vi "TestArmPathPlanner.vi"() -> ()   [LabVIEW 2018]
uses:
  TypeDefs/ArmAbsolutePosition.ctl
  General/MotionProfiling/TypeDefs/MotionProfileGeneratorParams.ctl
  <vilib>/Rock Robotics/WPI/ThirdParty/Phoenix-LabVIEW/Motor Controller/Controls/CTRE_Phoenix_MotorControl_TrajectoryPointTimeDur.ctl
  TypeDefs/ArmPassThroughParams.ctl
  TypeDefs/RobotID.ctl
  ArgosLib/Path Planning/TypeDefs/Point2D.ctl
  General/MotionProfiling/TypeDefs/TrajectoryPoint.ctl
  ArgosLib/ArgosLib.lvlib
panel:
  in  "PathPercent":dbl(slide) min=0.0 max=1.0 scale=0.0..1.0
  out "Arm Position":cluster{"X":dbl[], "Y":dbl[]}[](graph)=[{"X"=[-15.5, -15.5, -6.0, -6.0, 6.0, 6.0, 15.5, 15.5, 45.5, 45.5, 6.0, 6.0, -6.0, -6.0, -45.5, -45.5, -15.5], "Y"=[0.0, 7.0, 7.0, 12.0, 12.0, 7.0, 7.0, 0.0, 0.0, 90.0, 90.0, 24.0, 24.0, 90.0, 90.0, 0.0, 0.0]}, {"X"=array[361 elements], "Y"=array[361 elements]}, {"X"=array[361 elements], "Y"=array[361 elements]}, {"X"=[0.0, 21.000000000000004], "Y"=[44.25, 15.0]}, {"X"=[21.000000000000004, 26.99999809759101], "Y"=[15.0, 14.995222039735602]}, {"X"=[22.499999524397754, 22.499999524397758, 19.500000475602256, 19.500000475602253], "Y"=[14.9988055099339, 2.9988055099339004, 3.0011944900660996, 15.0011944900661]}]
  in  "Arm Pass Through Params":T1={"Pass Through Length (in)"=12.0, "Pass Through Min Height (in)"=12.0, "Pass Through Max Height (in)"=24.0, "Pass Through Wrist Angle (rad)"=0.0}
  out "Arm Wrist":T2(graph)={0.0, "Trajectory Point Interval (ms)"=40, [[4.055897027348257, 4.0550953656373006, 4.052237232134716, 4.04613843318791, 4.034997591857871, 4.015899135122442, 3.9848675439678005, 3.9367206365092895, 3.8639563502761987, 3.755694393958681, 3.5953226370164195, 3.360426119927916, 2.9841364514203983, 2.5860313232788723, 2.1668910532018417, 1.7245198623311084, 1.2463662836528413, 0.7434064615242622, 0.3302693816975075, 0.08764821007316621, -0.19010567504352455, -0.4928479002364374, -0.8053552192393434, -1.2552038154588934, -1.758124246438066, -2.287000533586975, -2.8485912983693416, -3.4544278992698296, -3.9992385919893625, -4.477495883282476, -4.902108995690553, -5.245537269018449, -5.245537269018449, -5.245537269018449, -5.245537269018449, -5.245537269018449, -5.245537269018449, -5.245537269018449, -5.245537269018449, -5.245537269018449, -5.245537269018449], [163.54485136741283, -0.020041542773907572, -0.0714533375646198, -0.15246997367013293, -0.2785210332509891, -0.4774614183857162, -0.7757897788660428, -1.2036726864627756, -1.819107155827271, -2.7065489079379446, -4.009293923556534, -5.872412927212589, -9.407241712687942, -9.952628203538149, -10.478506751925764, -11.059279771768331, -11.953839466956678, -12.573995553214479, -10.328426995668865, -6.065529290608533, -6.943847127917269, -7.5685556298228205, -7.81268297507265, -11.246214905488749, -12.573010774479314, -13.221907178722725, -14.039769119559164, -15.145915022512202, -13.620267317988322, -11.956432282327834, -10.615327810201935, -8.585706833197392, 0.0, 0.0, 0.0, 0.0, 0.0, 0.0, 0.0, 0.0, 0.0], [4088.6212841853207, -4089.122322754668, -1.2852948697678057, -2.0254159026378282, -3.151276489521404, -4.973509628368178, -7.458209012008165, -10.697072689918318, -15.385861734112382, -22.18604380276684, -32.56862539046473, -46.57797509140138, -88.3707196368838, -13.634662271255182, -13.146963709690374, -14.519325496064184, -22.363992379708673, -15.503902156445015, 56.13921393864034, 106.57244262650829, -21.95794593271838, -15.617712547638796, -6.103183631245734, -85.83829826040248, -33.169896724764136, -16.22241010608527, -20.446548520910966, -27.653647573825957, 38.141192613097004, 41.595875891512215, 33.52761180314747, 50.74052442511356, 214.6426708299348, 0.0, 0.0, 0.0, 0.0, 0.0, 0.0, 0.0, 0.0]]}
  out "Arm Shoulder":T2(graph)={0.0, "Trajectory Point Interval (ms)"=40, [[-2.485897027348257, -2.4851072958162197, -2.4823169806359386, -2.476610959105788, -2.466857228156793, -2.4515085113917974, -2.4287729667025824, -2.3963527600398518, -2.350431137808563, -2.284513709864505, -2.187157401405465, -2.040243693099315, -1.786824197239345, -1.5209887802060515, -1.2482788401614453, -0.9732781561615349, -0.6982771787555206, -0.4515858882028595, -0.3049850740385021, -0.10226983612994925, 0.11683754563303896, 0.3154399571329603, 0.4793394777948856, 0.7278750207432971, 1.0028758829523126, 1.2778768678302974, 1.5482951319817302, 1.8072546515485026, 1.9888767348636507, 2.1090685590963103, 2.1917192749834253, 2.2455372690184494, 2.2455372690184494, 2.2455372690184494, 2.2455372690184494, 2.2455372690184494, 2.2455372690184494, 2.2455372690184494, 2.2455372690184494, 2.2455372690184494, 2.2455372690184494], [0.0, 0.01974328830093297, 0.06975787950702639, 0.1426505382537635, 0.24384327372487524, 0.38371791912489295, 0.5683886172303754, 0.810505166568265, 1.1480405557822149, 1.6479356986014548, 2.433907711476002, 3.672842707653745, 6.335487396499251, 6.645885425832337, 6.817748501115156, 6.87501709999776, 6.875024435150356, 6.167282263816529, 3.6650203541089343, 5.067880947713822, 5.477684544074705, 4.965060287498034, 4.097488016548133, 6.213388573710287, 6.875021555225386, 6.875024621949621, 6.760456603785819, 6.473987989169311, 4.540552082878701, 3.0047956058164904, 2.066267897177876, 1.3454498508756019, 0.0, 0.0, 0.0, 0.0, 0.0, 0.0, 0.0, 0.0, 0.0], [0.0, 0.49358220752332427, 1.2503647801523354, 1.822316468668428, 2.5298183867777935, 3.4968661350004426, 4.616767452637061, 6.05291373344724, 8.438384730348746, 12.497378570480999, 19.649300321863684, 30.973374904443574, 66.56611722113765, 7.759950733327159, 4.29657688207048, 1.4317149720650901, 0.0001833788149108173, -17.69355428334569, -62.55654774268986, 35.071514840122184, 10.245089909022086, -12.815606414416791, -21.689306773747518, 52.897513929053865, 16.540824537877462, 7.666810588613515e-05, -2.864200454095056, -7.161715365412702, -48.33589765726525, -38.39391192655527, -23.463192715965363, -18.02045115755685, -33.636246271890045, 0.0, 0.0, 0.0, 0.0, 0.0, 0.0, 0.0, 0.0]]}
  out "Arm Extension":T2(graph)={0.0, "Trajectory Point Interval (ms)"=40, [[32.80243893371346, 32.73382329193226, 32.493830843461815, 32.014621982811256, 31.229704827724923, 30.07518621108094, 28.525539440458076, 26.595412909760075, 24.309668612420545, 21.71207960984723, 18.884301063490575, 16.058129522650766, 15.999999999999998, 15.999999999999998, 15.999999999999998, 15.999999999999998, 15.999999999999998, 17.018325645108163, 20.46619395704584, 20.10504894569543, 20.137290914005387, 20.263349380795905, 17.08862745921232, 15.999999999999998, 15.999999999999998, 15.999999999999998, 15.999999999999998, 15.999999999999998, 18.22509445834179, 20.899787030356347, 23.467846205438114, 25.612496949731394, 25.612496949731394, 25.612496949731394, 25.612496949731394, 25.612496949731394, 25.612496949731394, 25.612496949731394, 25.612496949731394, 25.612496949731394, 25.612496949731394], [0.0, -1.7153910445300014, -5.999811211761141, -11.980221516263967, -19.62292887715833, -28.862965416099584, -38.74116926557161, -48.25316326745001, -57.14360743348825, -64.93972506433288, -70.69446365891636, -70.65428852099522, -1.4532380662692024, 0.0, 0.0, 0.0, 0.0, 25.458141127704124, 86.19670779844188, -9.028625283760228, 0.8060492077489378, 3.151461669762945, -79.36804803958965, -27.21568648030801, 0.0, 0.0, 0.0, 0.0, 55.62736145854479, 66.86731430036392, 64.2014793770442, 53.616268607331996, 0.0, 0.0, 0.0, 0.0, 0.0, 0.0, 0.0, 0.0, 0.0], [0.0, -42.884776113250034, -107.11050418077849, -149.51025761257063, -191.06768402235906, -231.00091347353134, -246.95509623680056, -237.79985004696016, -222.2611041509559, -194.90294077111568, -143.86846486458714, 1.0043784480284756, 1730.0262613681502, 36.33095165673006, 0.0, 0.0, 0.0, 636.4535281926031, 1518.4641667684439, -2380.6333270550526, 245.86686228772913, 58.635311550350174, -2062.987742733815, 1303.809038982041, 680.3921620077002, 0.0, 0.0, 0.0, 1390.6840364636198, 280.9988210454781, -66.64587308299303, -264.63026924280496, -1340.4067151832999, 0.0, 0.0, 0.0, 0.0, 0.0, 0.0, 0.0, 0.0]]}
  out "Overall Motion":T2(graph)={0.0, "Trajectory Point Interval (ms)"=40, [[0.0, 0.07333333333333872, 0.32999999999999285, 0.8433333333333345, 1.6866666666666708, 2.933333333333337, 4.6200000000000045, 6.7466666666666715, 9.313333333333336, 12.320000000000004, 15.766666666666662, 19.577263128138455, 23.628890034857097, 27.882256707389793, 32.24561574810349, 36.645626692102056, 41.045642330598284, 45.23180493891788, 49.631804938917895, 53.752665022664445, 58.15266502266445, 62.15987106543, 66.55987106542999, 70.80102207008076, 75.20103586542501, 79.60105162347277, 83.92774384989569, 88.07109616296405, 91.88469944610591, 95.44136611277257, 98.59469944610589, 101.11264147745605, 101.11264147745605, 101.11264147745605, 101.11264147745605, 101.11264147745605, 101.11264147745605, 101.11264147745605, 101.11264147745605, 101.11264147745605, 101.11264147745605], [0.0, 1.8333333333334678, 6.416666666666354, 12.83333333333354, 21.083333333333407, 31.166666666666657, 42.166666666666686, 53.16666666666667, 64.16666666666661, 75.16666666666669, 86.16666666666646, 95.26491153679481, 101.29067266796605, 106.3341668133174, 109.0839760178424, 110.00027359996416, 110.0003909624057, 104.65406520798996, 110.00000000000031, 103.02150209366374, 110.00000000000014, 100.18015106913882, 109.9999999999996, 106.02877511626936, 110.00034488360626, 110.00039395119394, 108.16730566057302, 103.58380782670906, 95.34008207854647, 88.91666666666644, 78.83333333333304, 62.94855078375399, 0.0, 0.0, 0.0, 0.0, 0.0, 0.0, 0.0, 0.0, 0.0], [0.0, 45.8333333333367, 114.58333333332216, 160.41666666667965, 206.24999999999667, 252.08333333333127, 275.0000000000007, 274.99999999999966, 274.9999999999986, 275.00000000000176, 274.9999999999943, 227.45612175320886, 150.64402827928092, 126.08735363378365, 68.74523011312519, 22.90743955304393, 0.002934061038573077, -133.6581438603936, 133.64836980025885, -174.46244765841428, 174.46244765841, -245.49622327153315, 245.49622327151965, -99.2806220932561, 99.28924418342255, 0.0012266896920465342, -45.82720726552303, -114.58744584659897, -206.09314370406472, -160.58538529700073, -252.083333333335, -397.1195637394764, -1573.7137695938497, 0.0, 0.0, 0.0, 0.0, 0.0, 0.0, 0.0, 0.0]]}
  out "TravelTime (s)":dbl
  in  "MotionProfileGeneratorParameters":T3={"Trajectory Point Interval (ms)"=40, "Maximum Travel Speed (units/s)"=110.0, "Velocity Ramp Time (ms)"=400.0, "Acceleration Ramp Time (ms)"=200.0} {"Acceleration Ramp Time (ms)" min=1.0; "Velocity Ramp Time (ms)" min=1.0; "Maximum Travel Speed (units/s)" min=0.0; "Trajectory Point Interval (ms)" items=["TrajectoryDuration_0ms"=0, "TrajectoryDuration_5ms"=5, "TrajectoryDuration_10ms"=10, "TrajectoryDuration_20ms"=20, "TrajectoryDuration_30ms"=30, "TrajectoryDuration_40ms"=40, "TrajectoryDuration_50ms"=50, "TrajectoryDuration_100ms"=100]}
  in  "EndPoint":T5={"X (in)"=21.0, "Y (in)"=15.0, "Wrist (rad)"=1.57}
  in  "StartPoint":T5={"X (in)"=-18.0, "Y (in)"=50.0, "Wrist (rad)"=-1.0}
  in  "PathPointSpacing (in)":dbl=0.25
  out "PathLength (in)":dbl
  out "NumPoints":i32
  out "Path":cluster{dbl[], dbl[]}[](graph)=[{array[361 elements], array[361 elements]}, {array[361 elements], array[361 elements]}, {[-15.5, -15.5, -6.0, -6.0, 6.0, 6.0, 15.5, 15.5, 45.5, 45.5, 6.0, 6.0, -6.0, -6.0, -45.5, -45.5, -15.5], [0.0, 7.0, 7.0, 12.0, 12.0, 7.0, 7.0, 0.0, 0.0, 90.0, 90.0, 24.0, 24.0, 90.0, 90.0, 0.0, 0.0]}, {[-17.999999999999996, -17.969269066986136, -17.861710801437624, -17.64659427034059, -17.293188540681186, -17.23694880570164, -17.447845453869164, -17.482830899137877, -17.18187066722039, -16.361013245924966, -14.82948179588336, -12.47007247741721, -9.304518318749695, -6.95514637829422, -3.8898652435061973, 0.5101347564938068, 4.836801423160476, 8.558633631835997, 11.891422803105423, 14.941239308889699, 17.645200334636595, 19.97186447306996, 21.000000000000004, 21.000000000000004, 21.000000000000004, 21.000000000000004, 21.000000000000004, 21.000000000000004, 21.000000000000004, 21.000000000000004, 21.000000000000004], [50.0, 49.9334163118033, 49.70037340311485, 49.23428758573795, 48.468575171475905, 47.27284565759164, 45.60007000481347, 43.47500080506513, 40.928355772375475, 38.03974673892701, 34.95825798541716, 31.972081104358047, 29.42853115052185, 26.06948381963748, 24.0, 23.999999999999993, 23.999999999999993, 22.464819820898406, 20.465146318136746, 18.635256414666177, 17.01287979921804, 15.616881316158025, 15.0, 15.0, 15.0, 15.0, 15.0, 15.0, 15.0, 15.0, 15.0]}]
  out "Update Rate (Hz)":dbl
  in  "stop":bool
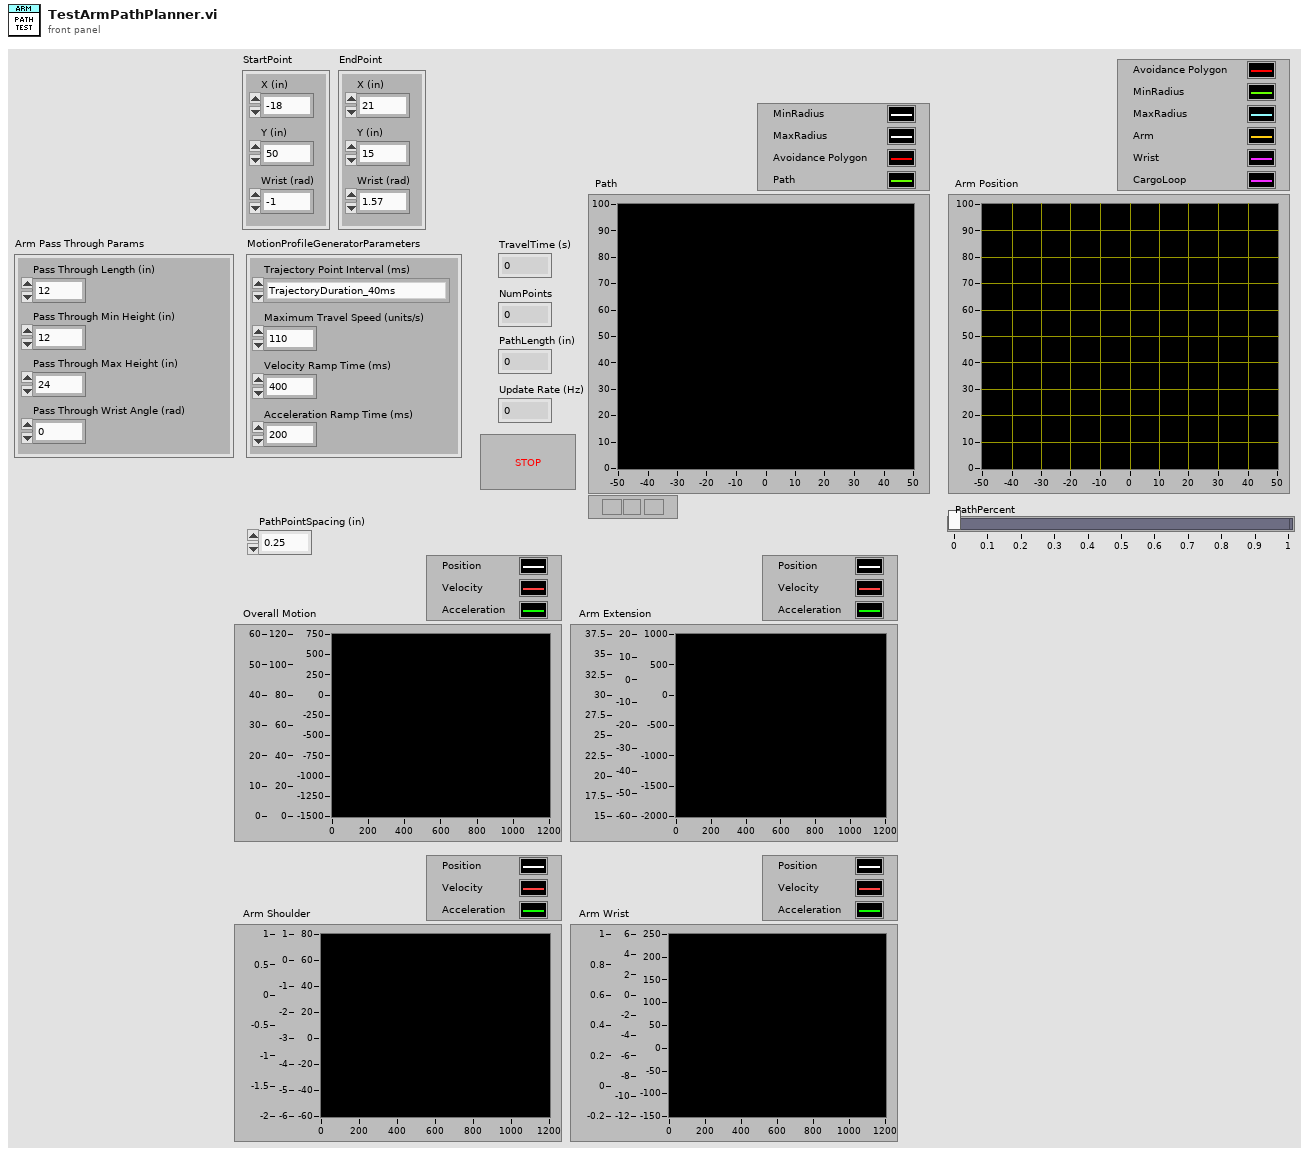
[diagram p1: front panel]
types:
  T1 = typedef "ArmPassThroughParams.ctl" = cluster{"Pass Through Length (in)":dbl, "Pass Through Min Height (in)":dbl, "Pass Through Max Height (in)":dbl, "Pass Through Wrist Angle (rad)":dbl}
  T2 = cluster{dbl, "Trajectory Point Interval (ms)":i32, dbl[][]}
  T3 = typedef "MotionProfileGeneratorParams.ctl" = cluster{"Trajectory Point Interval (ms)":T4, "Maximum Travel Speed (units/s)":dbl, "Velocity Ramp Time (ms)":dbl, "Acceleration Ramp Time (ms)":dbl}
  T4 = typedef "CTRE_Phoenix_MotorControl_TrajectoryPointTimeDur.ctl" = i32
  T5 = typedef "ArmAbsolutePosition.ctl" = cluster{"X (in)":dbl, "Y (in)":dbl, "Wrist (rad)":dbl}
  T6 = typedef "ArgosLib.lvlib/Point2D.ctl" = cluster{"X (in)":dbl, "Y (in)":dbl}
  T7 = typedef "RobotID.ctl" = enum16{"Competition", "Practice", "Programming"}
  T8 = typedef "TrajectoryPoint.ctl" = cluster{"Position ":dbl, "Velocity ":dbl, "Time (ms)":T4, "Last Point":bool}
  T9 = typedef "Config_Robot.ctl" = cluster{"Motors":cluster{"DriveRightPrimary":T10, "DriveRightSecondary":T10, "DriveLeftPrimary":T10, "DriveLeftSecondary":T10, "RearClimb":T10, "Front Climb":T10, "Climb Drive":T10, "Shoulder1":T10, "Shoulder2":T10, "Wrist":T10, "Extension":T10, "CargoIntake":T10, "Intake2":T10}, "Sensors":cluster{"IMU":T15, "HomingButton":T17, "HomingLED_Green":T17, "HomingLED_Yellow":T17, "HomingLED_Red":T17}, "PID":cluster{"FrontClimb":T19, "RearClimb":T19, "ArmShoulder":T19, "ArmExtend":T19, "ArmWrist":T19}, "Solenoids":cluster{" Shifter":T20, "Hatch Grip":T20, "Hatch Extend":T20, "Manipulator Slide":T20, "Hatch Floor Intake":T20}, "Enable Compressor":bool, "MotionMagic":cluster{"FrontClimbExtend":T22, "RearClimbExtend":T22, "FrontClimbRetract":T22, "RearClimbRetract":T22}, "RobotDimensions":T23, "Arm Home Position":T24, "Climb Home Position":cluster{"Back Climb":dbl, "Front Climb":dbl}, "Climb Positions":T25}
  T10 = typedef "ArgosLib.lvlib/Config_Motor.ctl" = cluster{"CAN Address":u8, "Invert":bool, "InvertSensor":bool, "Unit Conversion Factor":dbl, "Brake Mode":T11, "Reverse Limt Switch Mode":T12, "Forward Limt Swith Mode":T12, "PWM Channel":T13, "Motor Controller Type":T14, "Peak Current (A)":i32, "Continuos Current (A)":i32, "Peak Duration (ms)":i32, "Current Limit Enable":bool}
  T11 = typedef "CTRE_Phoenix_MotorControl_NeutralMode.ctl" = enum8{"EEPROMSetting", "Override to Coast", "Override to Brake"}
  T12 = typedef "CTRE_Phoenix_MotorControl_LimitSwitchNormal.ctl" = enum16{"Normally Open", "Normally Closed", "Disabled"}
  T13 = typedef "FPGA_DIOPWMChannel.ctl" = enum8{"PWM 0", "PWM 1", "PWM 2", "PWM 3", "PWM 4", "PWM 5", "PWM 6", "PWM 7", "PWM 8", "PWM 9", "PWM MXP 0", "PWM MXP 1", "PWM MXP 2", "PWM MXP 3", "PWM MXP 4", "PWM MXP 5", "PWM MXP 6", "PWM MXP 7", "PWM MXP 8", "PWM MXP 9", "Invalid"}
  T14 = typedef "ArgosLib.lvlib/Config_MotorCtrlType.ctl" = enum16{"Disabled", "Talon SRX", "Talon SR"}
  T15 = typedef "ArgosLib.lvlib/Config_IMU.ctl" = cluster{"Yaw Axis":enum16{"X", "Y", "Z"}, "SPI Bus":T16, "AHRS Algorithm":enum16{"Complementary", "Madgwick"}, "Calibration Time (s)":dbl, "Calibrate On Open":bool}
  T16 = typedef "spi_bus.ctl" = enum16{"SPI On-Board, CS0", "SPI On-Board, CS1", "SPI On-Board, CS2", "SPI On-Board, CS3", "SPI MXP", "Invalid"}
  T17 = typedef "ArgosLib.lvlib/Config_DigitalIO.ctl" = cluster{"DIOChannel":T18, "Active Low":bool}
  T18 = typedef "FPGA_DIOChannel.ctl" = enum8{"DIO 0", "DIO 1", "DIO 2", "DIO 3", "DIO 4", "DIO 5", "DIO 6", "DIO 7", "DIO 8", "DIO 9", "DIO MXP 0", "DIO MXP 1", "DIO MXP 2", "DIO MXP 3", "DIO MXP 4", "DIO MXP 5", "DIO MXP 6", "DIO MXP 7", "DIO MXP 8", "DIO MXP 9", "DIO MXP 10", "DIO MXP 11", "DIO MXP 12", "DIO MXP 13", "DIO MXP 14", "DIO MXP 15", "SPI Port CS1", "SPI Port CS2", "SPI Port CS3", "SPI Port MISO", "SPI Port MOSI", "Invalid"}
  T19 = typedef "ArgosLib.lvlib/Config_PIDParams.ctl" = cluster{"P":dbl, "I":dbl, "D":dbl, "F":dbl, "IZone":dbl}
  T20 = typedef "ArgosLib.lvlib/Config_SingleSolenoid.ctl" = cluster{"SolenoidChannel":T21, "Invert":bool}
  T21 = typedef "WPI_SolenoidChannel.ctl" = enum8{"Solenoid 0", "Solenoid 1", "Solenoid 2", "Solenoid 3", "Solenoid 4", "Solenoid 5", "Solenoid 6", "Solenoid 7", "Invalid"}
  T22 = typedef "Config_MotionMagicParams.ctl" = cluster{"CruiseVelocity":i32, "Acceleration":i32}
  T23 = typedef "Config_Dimensions.ctl" = cluster{"Length (in)":dbl, "Shoulder Height (in)":dbl, "Frame Height (in)":dbl, "Arm Center to Front of Robot (in)":dbl, "Arm Min Extension (in)":dbl, "Arm Max Extension (in)":dbl, "Cargo Intake Loop Length (in)":dbl, "Cargo Intake Loop Width (in)":dbl, "Cargo Intake Loop Offset (in)":dbl, "Cargo Intake Loop Angle (rad)":dbl}
  T24 = typedef "ArmCoordinate.ctl" = cluster{"Radius (in)":dbl, "ShoulderAngle (rad)":dbl, "WristAngle (rad)":dbl}
  T25 = typedef "ClimberPositionHeights.ctl" = cluster{"Retract":dbl, "Level 2":dbl, "Level 3":dbl}
  T26 = typedef "ArgosLib.lvlib/Polygon2D.ctl" = T6[]
  T27 = cluster{dbl, "Trajectory Point Interval (ms)":T4, dbl[][]}
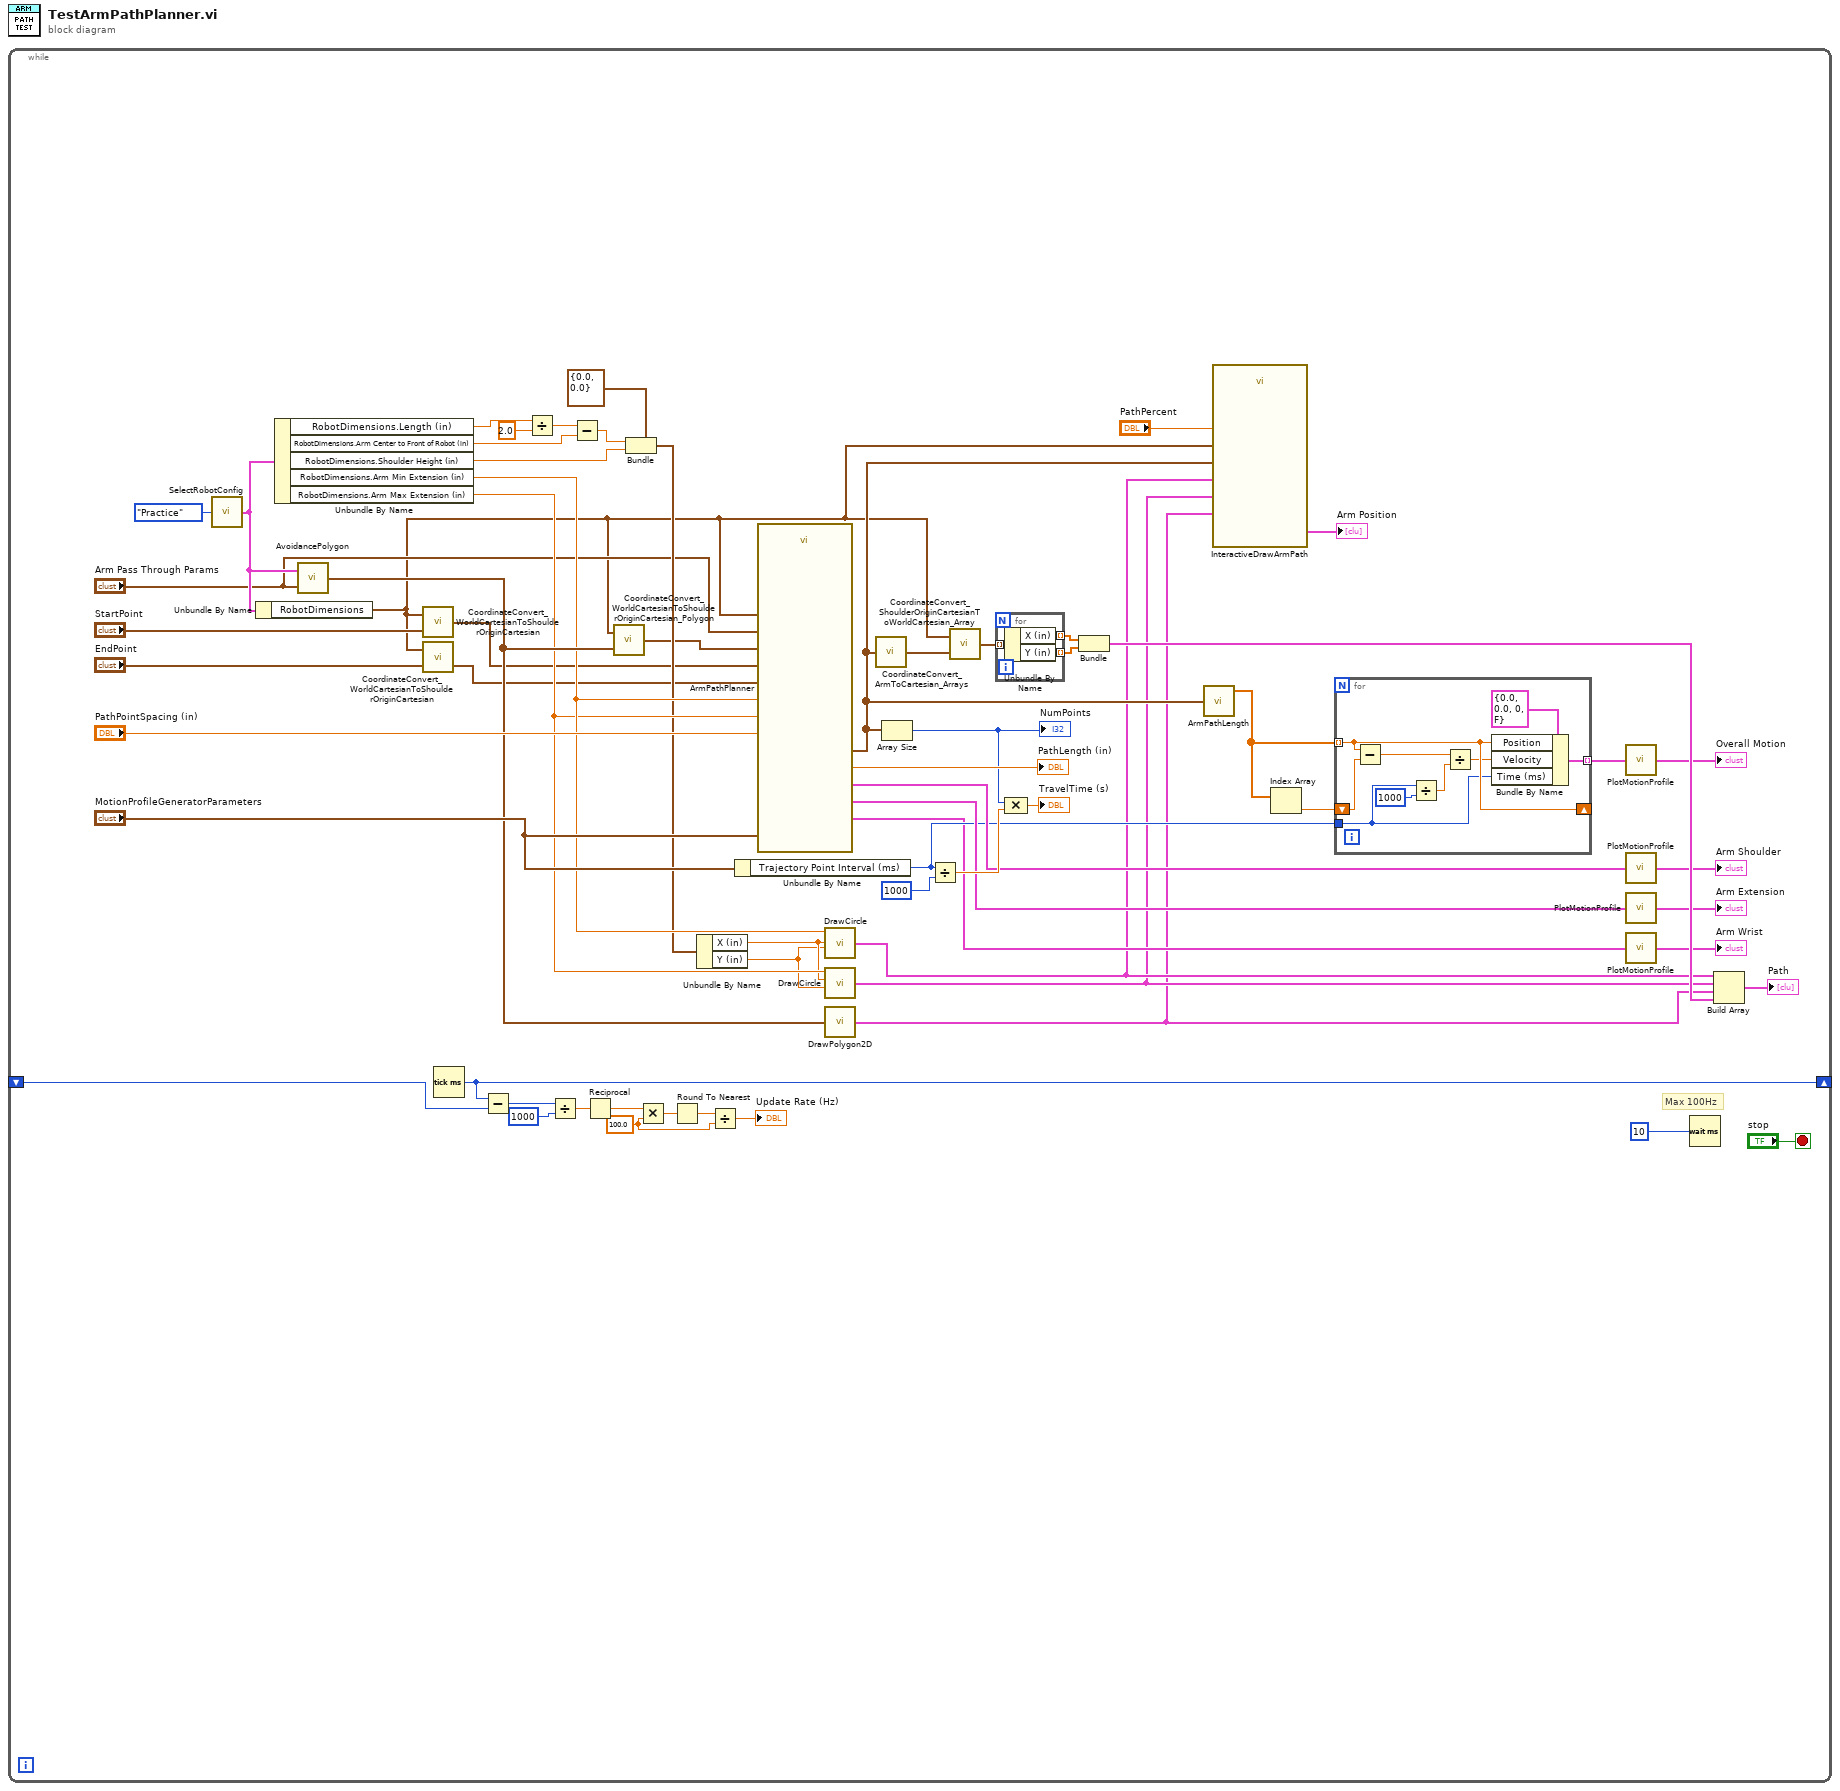
[diagram p0: block diagram]
diagram:
  n1 = while {
    shift-right: [w54] -> _
    shift-left: _ -> [w55]
    stop <- "stop" stop-if-true
    w57 = 100.0 ("y")
    # "Max 100Hz"
    n2 = call "SelectRobotConfig.vi"("Robot ID"=RobotID."Practice") -> ("Selected Config"=w8:T9)
    n3 = Unbundle By Name(w8) -> ("RobotDimensions"=w1:T23)
    n4 = Unbundle By Name(w8) -> ("RobotDimensions.Length (in)"=w22:dbl, "RobotDimensions.Arm Center to Front of Robot (in)"=w19:dbl, "RobotDimensions.Shoulder Height (in)"=w16:dbl, "RobotDimensions.Arm Min Extension (in)"=w13:dbl, "RobotDimensions.Arm Max Extension (in)"=w12:dbl)
    n5 = call "AvoidancePolygon.vi"("Arm Pass Through Params"="Arm Pass Through Params", "RobotConfig"=w8) -> ("Polygon"=w30:T26)
    n6 = call "CoordinateConvert_WorldCartesianToShoulderOriginCartesian.vi"("ArmPositionIn"="StartPoint", "RobotDimensions"=w1) -> ("ArmPositionRelativeToShoulder"=w6:T5)
    n7 = call "CoordinateConvert_WorldCartesianToShoulderOriginCartesian.vi"("ArmPositionIn"="EndPoint", "RobotDimensions"=w1) -> ("ArmPositionRelativeToShoulder"=w5:T5)
    n8 = Tick Count (ms)() -> (millisecond timer value=w54:u32)
    n9 = Subtract(x=w54, y=w55) -> (x-y=w63:u32)
    n10 = Divide(x=w22, y=2.0) -> (x/y=w20:dbl)
    n11 = Divide(x=w63, y=u32 1000) -> (x/y=w61:dbl)
    n12 = Subtract(x=w20, y=w19) -> (x-y=w17:dbl)
    n13 = Reciprocal(x=w61) -> (1/x=w60:dbl)
    n14 = call "CoordinateConvert_WorldCartesianToShoulderOriginCartesian_Polygon.vi"("ArmPositionIn"=w30, "RobotDimensions"=w1) -> ("ArmPositionRelativeToShoulder"=w3:T26)
    n15 = Bundle(cluster=T6 {"X (in)"=0.0, "Y (in)"=0.0} ("2DPoint"), "X (in)"=w17, "Y (in)"=w16) -> (w11:T6)
    n16 = Multiply(x=w60, y=w57) -> (x*y=w59:dbl)
    n17 = Round To Nearest(number=w59) -> (nearest integer value=w58:dbl)
    n18 = Unbundle By Name(w11) -> ("X (in)"=w10:dbl, "Y (in)"=w9:dbl)
    n19 = Divide(x=w58, y=w57) -> (x/y=→"Update Rate (Hz)":dbl)
    n20 = Unbundle By Name("MotionProfileGeneratorParameters") -> ("Trajectory Point Interval (ms)"=w33:T4)
    n21 = call "ArmPathPlanner.vi"("StartPoint"=w6, "EndPoint"=w5, "PathPointSpacing (in)"="PathPointSpacing (in)", "MinArmLength"=w13, "MaxArmLength"=w12, "AvoidancePolygon"=w3, "RobotDimensions"=w1, "MotionProfileGeneratorParameters"="MotionProfileGeneratorParameters", "Arm Pass Through Params"="Arm Pass Through Params") -> ("Path"=w26:T24[], "ShoulderPath"=w37:T8[], "ExtendPath"=w36:T8[], "WristPath"=w28:T8[], "PathLength (in)"=→"PathLength (in)":dbl)  [unwired: 6 in]
    n22 = call "DrawCircle.vi"("YCenter"=w9, "XCenter"=w10, "Radius"=w13) -> ("Points"=w25:cluster{"X":dbl[], "Y":dbl[]})  [unwired: 1 in]
    n23 = call "DrawCircle.vi"("YCenter"=w9, "XCenter"=w10, "Radius"=w12) -> ("Points"=w24:cluster{"X":dbl[], "Y":dbl[]})  [unwired: 1 in]
    n24 = call "DrawPolygon2D.vi"("Polygon"=w30) -> ("XYPlot"=w23:cluster{dbl[], dbl[]})
    n25 = call "CoordinateConvert_ArmToCartesian_Arrays.vi"("ArmCoordinates"=w26) -> ("XYPoints"=w51:T5[])
    n26 = Array Size(array=w26) -> (size(s)=w42:i32)
    "NumPoints" <- w42
    n27 = Divide(x=w33, y=1000) -> (x/y=w40:dbl)
    n28 = call "CoordinateConvert_ShoulderOriginCartesianToWorldCartesian_Array.vi"("ArmPositionRelativeToShoulderIn"=w51, "RobotDimensions"=w1) -> ("ArmAbsolutePosition"=w4:T5[])
    n29 = for {
      tunnel: w4 -> [w76] mode=indexing
      tunnel: [w75] -> w50 mode=indexing
      tunnel: [w74] -> w49 mode=indexing
      n30 = Unbundle By Name(w76) -> ("X (in)"=w75:dbl, "Y (in)"=w74:dbl)
    }
    n31 = Compound Arithmetic op=MULTIPLY(w42, w40) -> (→"TravelTime (s)":dbl)
    n32 = Bundle(w50, w49) -> (w47:cluster{dbl[], dbl[]})  [unwired: 1 in]
    n33 = call "ArmPathLength.vi"("ArmPathIn"=w26) -> ("IndexedPathLength"=w32:dbl[])  [unwired: 2 in, 2 out]
    n34 = call "InteractiveDrawArmPath.vi"("PathPercent"="PathPercent", "RobotDimensions"=w1, "AvoidancePolygon"=w23, "MaxRadiusCircle"=w24, "MinRadiusCircle"=w25, "Path"=w26) -> ("Arm Position"=→"Arm Position":cluster{"X":dbl[], "Y":dbl[]}[])  [unwired: 5 in]
    n35 = Index Array(array=w32) -> (element=w31:dbl)  [unwired: 1 in]
    n36 = for {
      tunnel: [w72] -> w34 mode=indexing
      tunnel: w32 -> [w71] mode=indexing
      tunnel: w33 -> [w69]
      shift-right: [w71] -> _
      shift-left: w31 -> [w70]
      n37 = Subtract(x=w71, y=w70) -> (x-y=w67:dbl)
      n38 = Divide(x=w69, y=1000) -> (x/y=w66:dbl)
      n39 = Divide(x=w67, y=w66) -> (x/y=w65:dbl)
      n40 = Bundle By Name(cluster=T8 {"Position "=0.0, "Velocity "=0.0, "Time (ms)"=0, "Last Point"=FALSE} ("trajectory point"), "Position"=w71, "Velocity"=w65, "Time (ms)"=w69) -> (w72:T8)
    }
    n41 = call "PlotMotionProfile.vi"("Trajectory Points"=w34) -> ("MotionProfileGraph"=→"Overall Motion":T27)
    n42 = call "PlotMotionProfile.vi"("Trajectory Points"=w37) -> ("MotionProfileGraph"=→"Arm Shoulder":T27)
    n43 = call "PlotMotionProfile.vi"("Trajectory Points"=w36) -> ("MotionProfileGraph"=→"Arm Extension":T27)
    n44 = call "PlotMotionProfile.vi"("Trajectory Points"=w28) -> ("MotionProfileGraph"=→"Arm Wrist":T27)
    n45 = Wait (ms)(milliseconds to wait=u32 10) -> ()  [unwired: 1 out]
    n46 = Build Array(w25, w24, w23, w47) -> (→"Path":cluster{"X":dbl[], "Y":dbl[]}[])
  }
